vi "myRIO v1.0 Unreserve AudioIn Block.vi"(7 "Allow multiple opens?":bool, 8 "error in (no error)":errorcluster, 10 "AudioIn (N Samples) Channel List":T1) -> (0 "error out":errorcluster)   [LabVIEW 2021]
uses:
  <vilib>/myRIO/Common/Instrument Driver Framework/myRIO v1.0/AudioIn Block/typedefs/AudioIn Block Channels List.ctl
  <vilib>/myRIO/Common/Instrument Driver Framework/myRIO v1.0/AudioIn Block/typedefs/AudioIn Block Channels Enum.ctl
  <vilib>/myRIO/Common/Instrument Driver Framework/myRIO v1.0/Resource Manager/vis/myRIO v1.0 Unreserve Channel.vi
  <vilib>/myRIO/Common/Instrument Driver Framework/myRIO v1.0/Resource Manager/vis/myRIO v1.0 Build Mutex Name.vi
  <vilib>/myRIO/Common/Instrument Driver Framework/Utilities/vis/Configuration Manager.vi
  <vilib>/myRIO/Common/Instrument Driver Framework/Utilities/vis/IO Manager.vi
  <vilib>/Utility/error.llb/Error Cluster From Error Code.vi
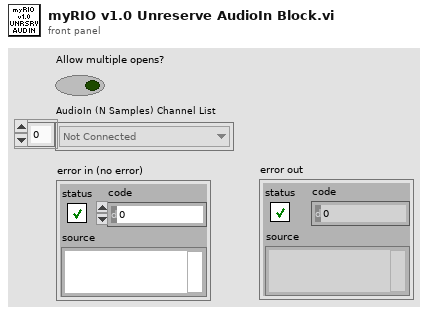
[diagram p1: front panel]
types:
  T1 = typedef "AudioIn Block Channels List.ctl" = T2[]
  T2 = typedef "AudioIn Block Channels Enum.ctl" = enum16{"Not Connected", "AudioIn/Left (N Samples)", "AudioIn/Right (N Samples)"}
  T3 = typedef "myRIO v1.0 Channel Reservation List.ctl" = T4[]
  T4 = typedef "myRIO v1.0 Channel Reservation Info.ctl" = cluster{"Channel Name":string, "Connector":T5, "Mutex ID":i32}
  T5 = typedef "myRIO v1.0 Connector List.ctl" = enum32{"None", "ConnectorA", "ConnectorB", "ConnectorC"}
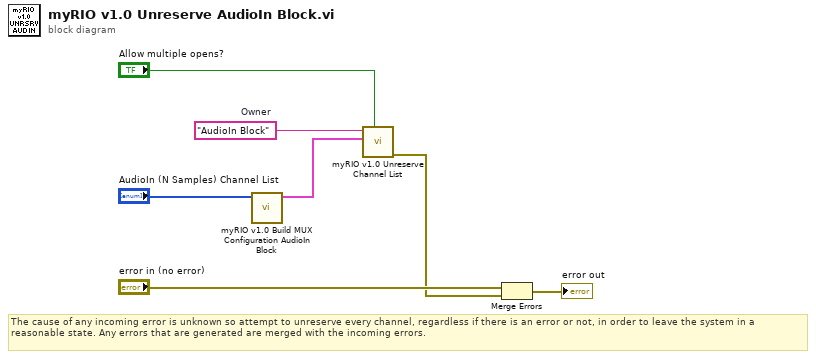
[diagram p0: block diagram]
diagram:
  w2 = "AudioIn Block"  # Owner
  # "The cause of any incoming error is unknown so attempt to unreserve every channel, regardless if there is an error or not, in order to leave the system in a reasonable state. Any errors that are generated are merged with the incoming errors."
  n1 = call <vilib>:"myRIO v1.0 Build MUX Configuration AudioIn Block.vi"("AudioIn (N Samples) Channels List"="AudioIn (N Samples) Channel List") -> ("Channel Reservation Info"=w3:T3)  [unwired: 10 in]
  n2 = call <vilib>:"myRIO v1.0 Unreserve Channel List.vi"("Allow multiple opens?"="Allow multiple opens?", "Channel Reservation List"=w3, "Owner"=w2) -> ("error out"=w1:errorcluster)  [unwired: 8 in]
  n3 = Merge Errors("error in (no error)", w1) -> (→"error out":errorcluster)
